vi "MJG_trueCounter_v1.vi"(11 "True?":bool) -> (3 "True Count":u32)   [LabVIEW 2016]
panel:
  # ">>>"
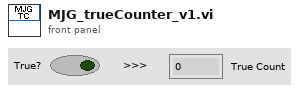
[diagram p1: front panel]
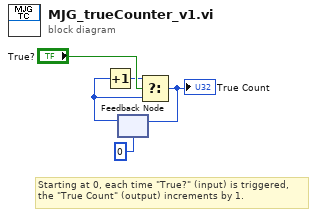
[diagram p0: block diagram]
diagram:
  # "Starting at 0, each time \"True?\" (input) is triggered, \nthe \"True Count\" (output) increments by 1."
  n1 = feedback #1(u32 0) -> (w2:u32)
  n2 = Increment(x=w2) -> (x+1=w4:u32)
  n3 = Select(t=w4, s="True?", f=w2) -> (s? t:f=w1:u32)
  "True Count" <- w1
  n4 = feedback-in #1(w1) -> ()
